vi "Booting.vi"() -> ()   [LabVIEW 2021]
uses:
  <vilib>/Utility/miscctls.llb/LVPointTypeDef.ctl
panel:
  out "Ring":u16(ring)
  # "Loading........"
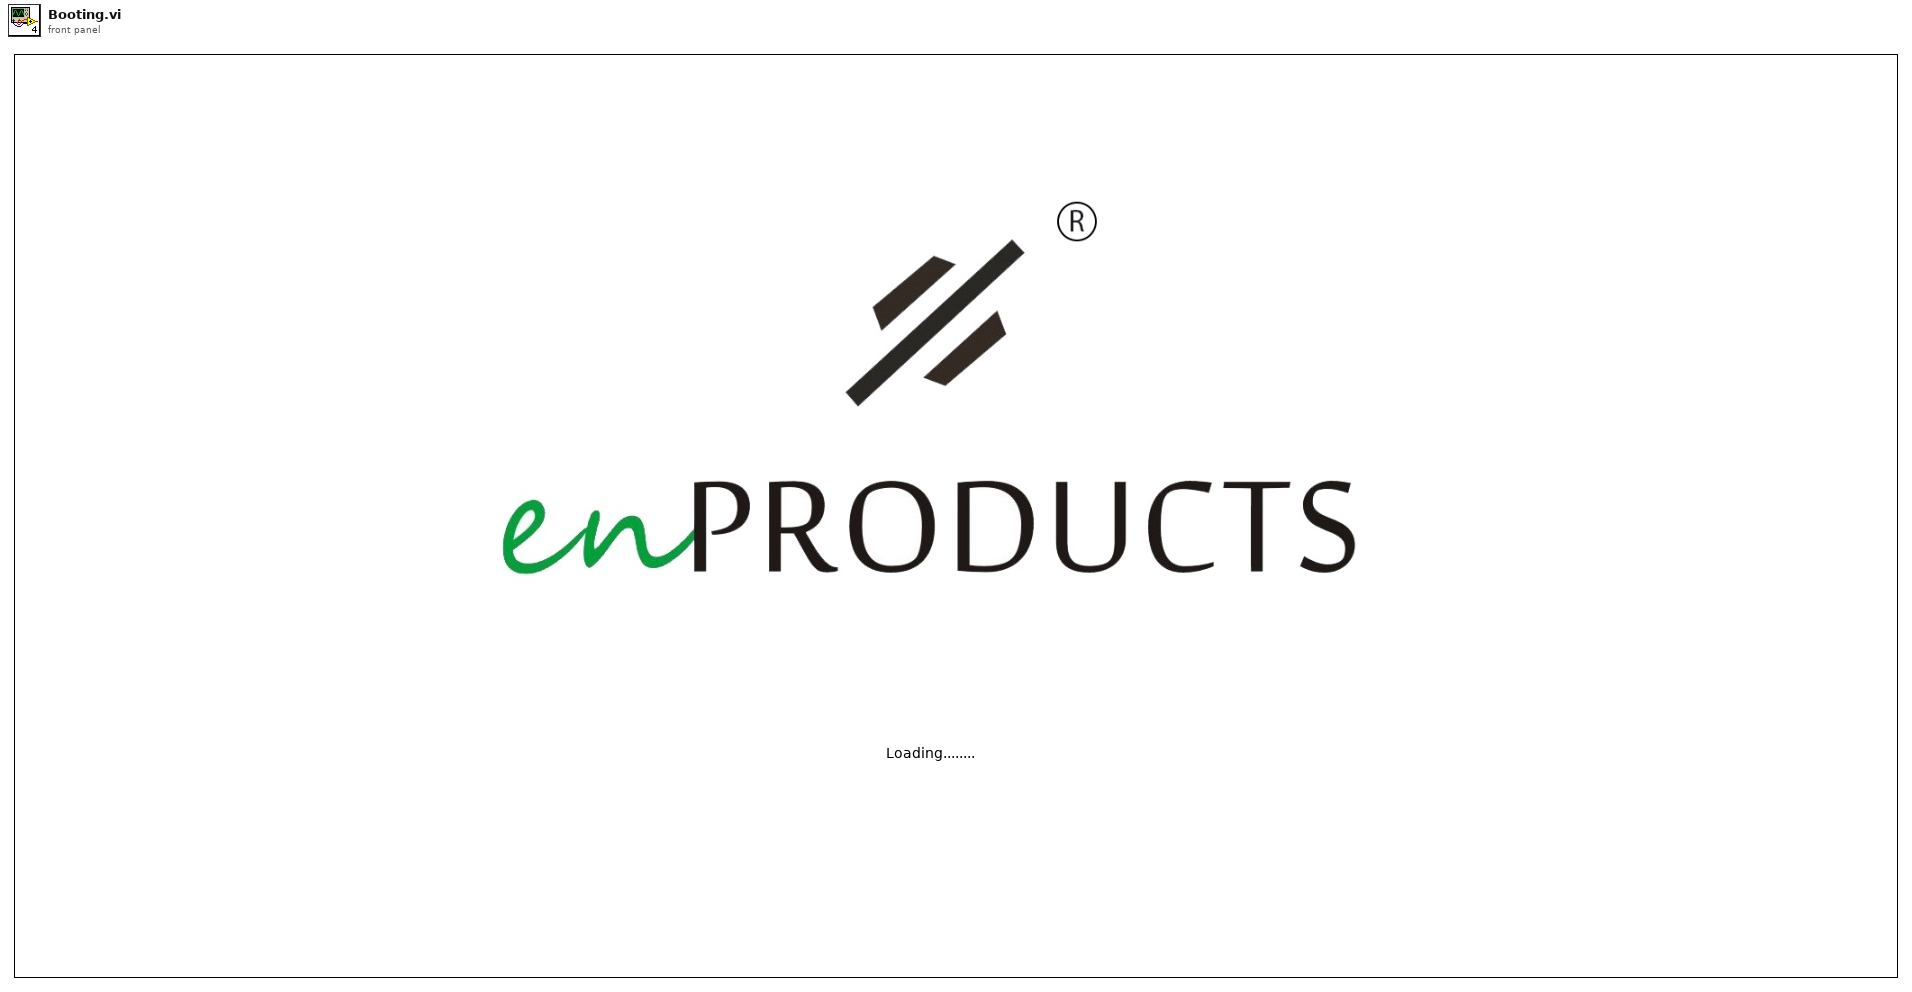
[diagram p1: front panel]
types:
  T1 = typedef "LVPointTypeDef.ctl" = cluster{"Horizontal":i16, "Vertical":i16}
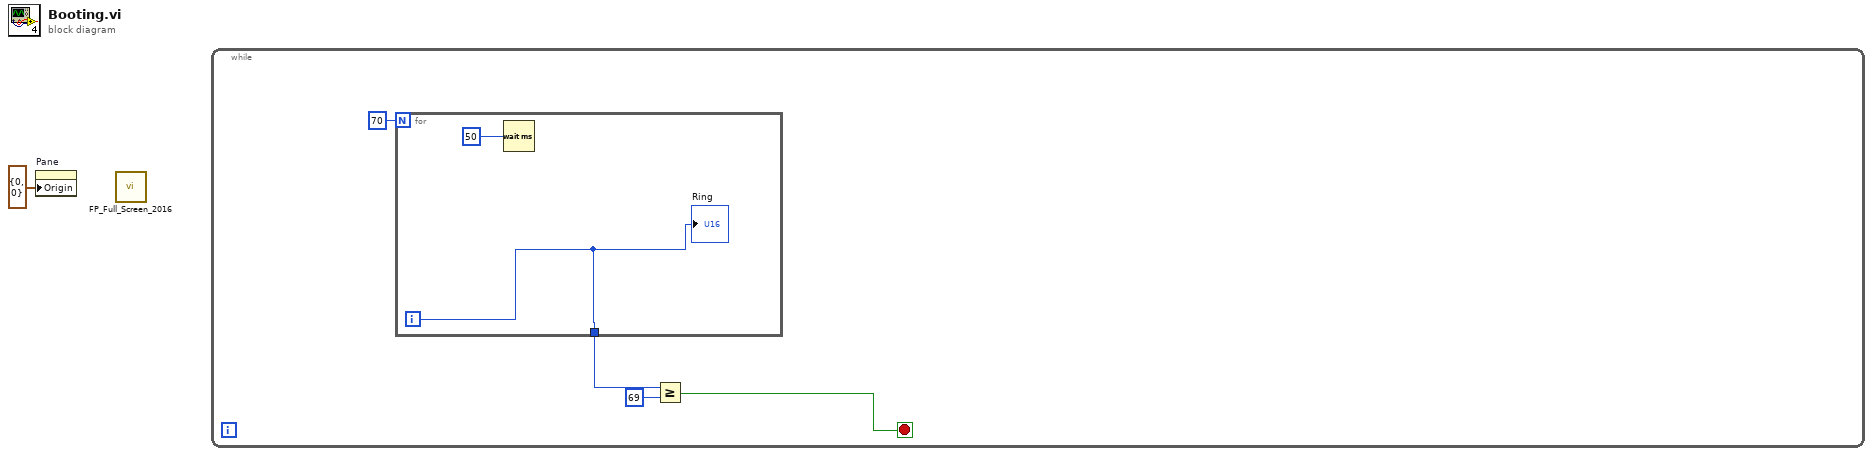
[diagram p0: block diagram]
diagram:
  n1 = property on="Pane" class="Pane"("Origin"=T1 {"Horizontal"=0, "Vertical"=0}) -> ()  [unwired: 2 in, 2 out]
  n2 = call "FP_Full_Screen_2016.vi"() -> ()  [unwired: 12 in]
  n3 = while {
    stop <- w3 stop-if-true
    n4 = for {
      N: 70 -> [_]
      tunnel: [w6] -> w4
      i -> [w6]
      n5 = Wait (ms)(milliseconds to wait=u32 50) -> ()  [unwired: 1 out]
      "Ring" <- w6
    }
    n6 = Greater Or Equal?(x=w4, y=69) -> (x >= y?=w3:bool)
  }
